vi "Configure Mode.vi"(8 "error in (no error)":errorcluster, 9 "Power-Up Mode (1: Active Mode)":u16(ring)=1 items=["Active Mode"=1, "Continuous Mode"=2, "Idle Mode"=3], 10 "Instrument Mode (1: Active Mode)":u16(ring)=1 items=["Active Mode"=1, "Continuous Mode"=2, "Idle Mode"=3, "Sleep Mode"=4, "Deep Sleep Mode"=5], 11 "VISA resource name":refnum<visa-resource-name>) -> (0 "error out":errorcluster, 3 "VISA resource name out":refnum<visa-resource-name>)   [LabVIEW 2012, in "MicroStrain 3DM-GXx.lvlib"]
doc: "Configures the current mode of the Attitude Heading and Reference Systems (AHRS). The VI also configures the desired mode upon device startup.\n\n<B>Note:</B>\n- The Sleep Modes are valid only when Serial connections are used to establish communication with the instrument."
uses:
  <instrlib>/MicroStrain 3DM-GXx/MicroStrain 3DM-GXx.lvlib
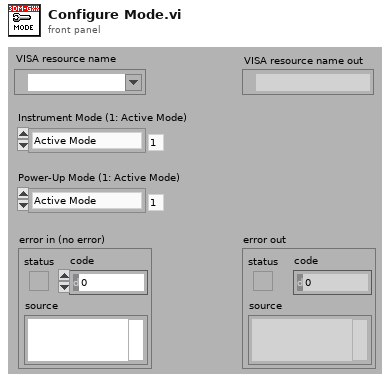
[diagram p1: front panel]
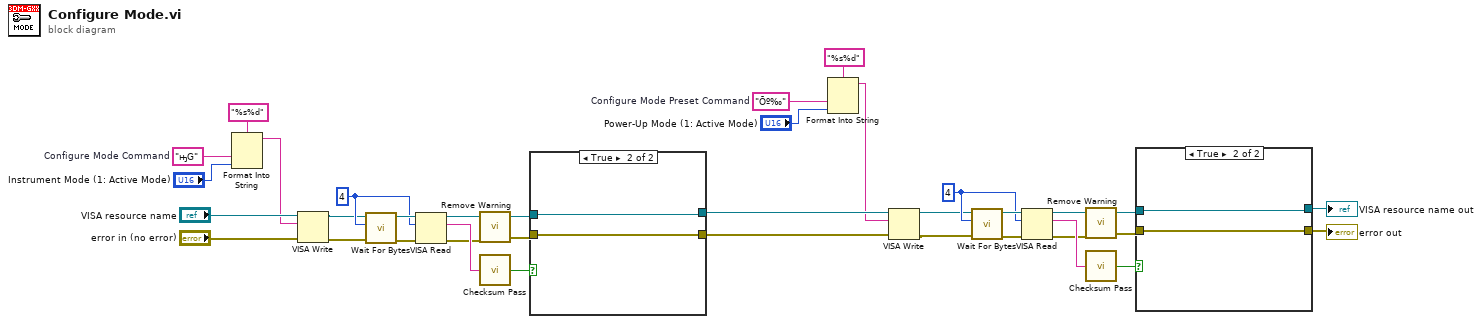
[diagram p0: block diagram]
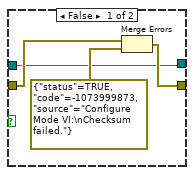
[diagram p2: hidden frame]
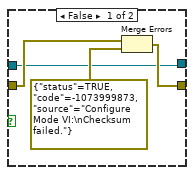
[diagram p3: hidden frame]
diagram:
  w11 = u32 4 ("Bytes To Read (0)")
  w17 = "Õº‰"  # Configure Mode Preset Command
  w28 = u32 4 ("Bytes To Read (0)")
  w34 = "ԣG"  # Configure Mode Command
  n1 = Format Into String(format string="%s%d", w34, "Instrument Mode (1: Active Mode)") -> (resulting string=w31:string)  [unwired: 2 in, 1 out]
  n2 = VISA Write(VISA resource name="VISA resource name", write buffer=w31, error in (no error)="error in (no error)") -> (VISA resource name out=w24:refnum<visa-resource-name>, error out=w23:errorcluster)  [unwired: 1 out]
  n3 = call <instrlib>:"Wait For Bytes.vi"("error in (no error)"=w23, "Bytes To Read (0)"=w28, "VISA resource name"=w24) -> ("error out"=w29:errorcluster, "VISA resource name out"=w30:refnum<visa-resource-name>)  [unwired: 7 in]
  n4 = VISA Read(VISA resource name=w30, byte count=w28, error in (no error)=w29) -> (VISA resource name out=w26:refnum<visa-resource-name>, read buffer=w27:string, error out=w25:errorcluster)  [unwired: 1 out]
  n5 = call <instrlib>:"Remove Warning.vi"("error in (no error)"=w25, "VISA resource name"=w26) -> ("error out"=w21:errorcluster, "VISA resource name out"=w22:refnum<visa-resource-name>)  [unwired: 2 in]
  n6 = call <instrlib>:"Checksum Pass.vi"("Message In"=w27) -> ("Checksum Pass"=w20:bool)  [unwired: 4 in]
  n7 = case shown="True" w20 {
    tunnel: w21 -> [w40 w42]
    tunnel: [w39 w42] -> w18
    tunnel: [w37 w41] -> w19
    tunnel: w22 -> [w37 w41]
    frame False {
      n8 = Merge Errors(w40, errorcluster {"status"=TRUE, "code"=-1073999873, "source"="Configure Mode VI:\nChecksum failed."} ("error in 2 (no error)")) -> (w39:errorcluster)
    }
    frame True {
    }
  }
  n9 = Format Into String(format string="%s%d", w17, "Power-Up Mode (1: Active Mode)") -> (resulting string=w14:string)  [unwired: 2 in, 1 out]
  n10 = VISA Write(VISA resource name=w19, write buffer=w14, error in (no error)=w18) -> (VISA resource name out=w4:refnum<visa-resource-name>, error out=w3:errorcluster)  [unwired: 1 out]
  n11 = call <instrlib>:"Wait For Bytes.vi"("error in (no error)"=w3, "Bytes To Read (0)"=w11, "VISA resource name"=w4) -> ("error out"=w12:errorcluster, "VISA resource name out"=w13:refnum<visa-resource-name>)  [unwired: 7 in]
  n12 = VISA Read(VISA resource name=w13, byte count=w11, error in (no error)=w12) -> (VISA resource name out=w9:refnum<visa-resource-name>, read buffer=w10:string, error out=w8:errorcluster)  [unwired: 1 out]
  n13 = call <instrlib>:"Remove Warning.vi"("error in (no error)"=w8, "VISA resource name"=w9) -> ("error out"=w6:errorcluster, "VISA resource name out"=w7:refnum<visa-resource-name>)  [unwired: 2 in]
  n14 = call <instrlib>:"Checksum Pass.vi"("Message In"=w10) -> ("Checksum Pass"=w5:bool)  [unwired: 4 in]
  n15 = case shown="True" w5 {
    tunnel: w6 -> [w46 w48]
    tunnel: [w45 w48] -> w2
    tunnel: [w43 w47] -> w1
    tunnel: w7 -> [w43 w47]
    frame False {
      n16 = Merge Errors(w46, errorcluster {"status"=TRUE, "code"=-1073999873, "source"="Configure Mode VI:\nChecksum failed."} ("error in 2 (no error)")) -> (w45:errorcluster)
    }
    frame True {
    }
  }
  "VISA resource name out" <- w1
  "error out" <- w2
